vi "pyCode close.vi"(8 "error in (no error)":errorcluster, 11 "pyCode in":refnum<class "pyCode.lvclass">) -> (0 "error out":errorcluster, 3 "pyCode out":refnum<class "pyCode.lvclass">)   [LabVIEW 2018, in "pyCode.lvclass"]
uses:
  pyCode.lvclass
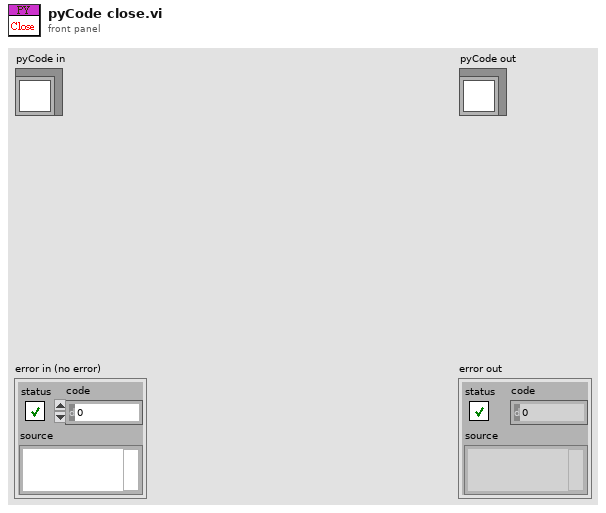
[diagram p1: front panel]
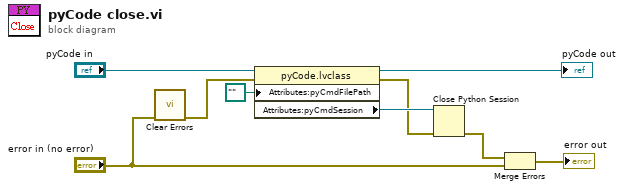
[diagram p0: block diagram]
diagram:
  n1 = call <vilib>:"Clear Errors.vi"("error in (no error)"="error in (no error)") -> ("error out"=w4:errorcluster)  [unwired: 5 in, 1 out]
  n2 = property class="pyCode.lvclass"(reference="pyCode in", error in=w4, "Attributes:pyCmdFilePath"=path "" ("pyCmdFilePath")) -> (reference out=→"pyCode out":refnum<class "pyCode.lvclass">, error out=w5:errorcluster, "Attributes:pyCmdSession"=w6:refnum<k35>)
  n3 = Close Python Session(session in=w6, error in=w5) -> (11:w3:errorcluster)
  n4 = Merge Errors(w3, "error in (no error)") -> (→"error out":errorcluster)
